vi "Insert.vi"(4 "da":dbl, 6 "iy":i32, 7 "dy weight":dbl, 9 "ix":i32, 10 "dx":dbl[](array[numeric]), 11 "dy in":dbl[](array[numeric])) -> (3 "dy out":dbl[](array[numeric]))   [LabVIEW 2014]
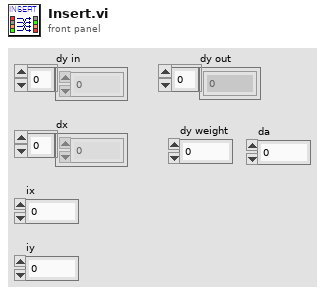
[diagram p1: front panel]
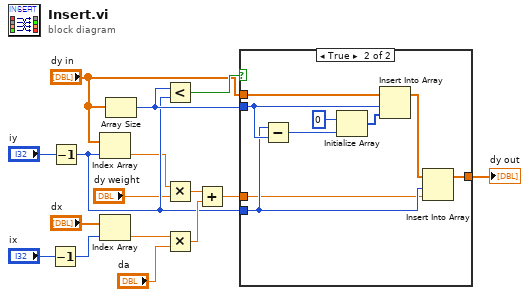
[diagram p0: block diagram]
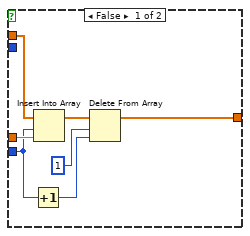
[diagram p2: hidden frame]
diagram:
  n1 = Decrement(x="ix") -> (x-1=w13:i32)
  n2 = Decrement(x="iy") -> (x-1=w5:i32)
  n3 = Index Array(array="dy in", index=w5) -> (element=w4:dbl)
  n4 = Index Array(array="dx", index=w13) -> (element=w14:dbl)
  n5 = Array Size(array="dy in") -> (size(s)=w15:i32)
  n6 = Less?(x=w15, y=w5) -> (x < y?=w11:bool)
  n7 = Multiply(x=w4, y="dy weight") -> (x*y=w1:dbl)
  n8 = Multiply(x=w14, y="da") -> (x*y=w8:dbl)
  n9 = Add(x=w1, y=w8) -> (x+y=w2:dbl)
  n10 = case shown="True" w11 {
    tunnel: "dy in" -> [w23 w24]
    tunnel: w2 -> [w22 w26]
    tunnel: w5 -> [w18 w27]
    tunnel: [w20 w25] -> w16
    tunnel: w15 -> [_ w29]
    frame False {
      n11 = Increment(x=w18) -> (x+1=w17:i32)
      n12 = Insert Into Array(array=w23, index=w18, new element=w22) -> (w21:dbl[])
      n13 = Delete From Array(array=w21, length=1, index=w17) -> (array with subset deleted=w20:dbl[])  [unwired: 1 out]
    }
    frame True {
      n14 = Subtract(x=w27, y=w29) -> (x-y=w30:i32)
      n15 = Initialize Array(0 ("element"), w30) -> (w31:i32[])
      n16 = Insert Into Array(array=w24, index=w29, new element=w31) -> (w28:dbl[])
      n17 = Insert Into Array(array=w28, index=w27, new element=w26) -> (w25:dbl[])
    }
  }
  "dy out" <- w16
